vi "GetSimWAVFile.vi"(8 "error in (no error)":errorcluster) -> (0 "error out":errorcluster, 3 "wav file path":path)   [LabVIEW 2017, in "EmsaAudio.lvlib"]
uses:
  <vilib>/addons/InsightCM/Devices/Shared/Emsa/EmsaAudio/EmsaAudio.lvlib
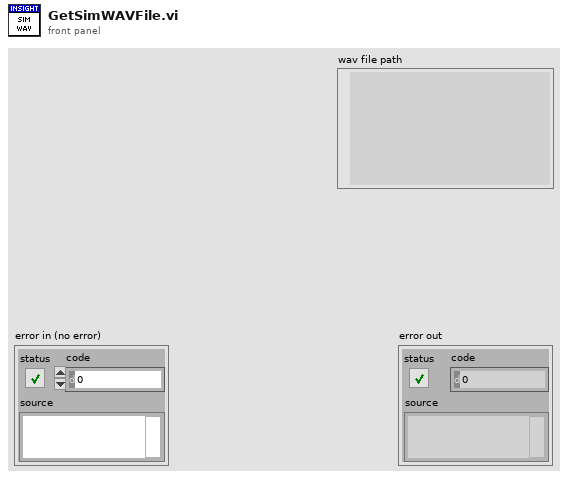
[diagram p1: front panel]
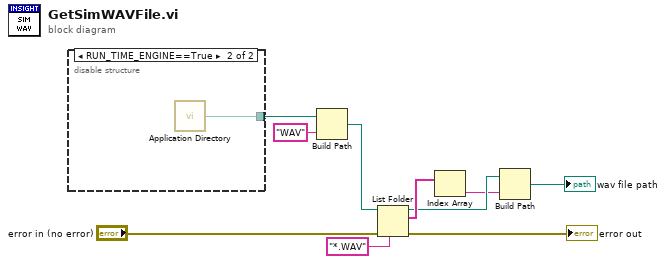
[diagram p0: block diagram]
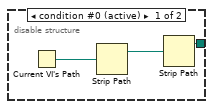
[diagram p2: hidden frame]
diagram:
  n1 = disable-structure shown="RUN_TIME_ENGINE==True" {
    disable-tunnel: [w11 w14] -> w10
    frame condition #0 (active) {
      n2 = Current VI's Path() -> (path=w13:path)
      n3 = Strip Path(path=w13) -> (stripped path=w12:path)  [unwired: 1 out]
      n4 = Strip Path(path=w12) -> (stripped path=w11:path)  [unwired: 1 out]
    }
    frame condition #1 {
      n5 = call <vilib>:"Application Directory.vi"() -> ("Application Directory"=w14:path)
    }
  }
  n6 = Build Path(base path=w10, name or relative path="WAV") -> (appended path=w8:path)
  n7 = List Folder(path=w8, pattern="*.WAV", error in="error in (no error)") -> (path out=w3:path, filenames=w4:string[], error out=→"error out":errorcluster)  [unwired: 1 in, 1 out]
  n8 = Index Array(array=w4) -> (element=w2:string)  [unwired: 1 in]
  n9 = Build Path(base path=w3, name or relative path=w2) -> (appended path=→"wav file path":path)
